vi "Begin.vi"(8 "error in":errorcluster) -> (0 "error out":errorcluster)   [LabVIEW 2019]
doc: "Called before other user functions, this VI is expected to open initial I/O refnums, load in file data, and do all program initialization. Notice that the <B>error out</B> terminal is simply used for data flow. Wiring it to other structures or subVIs ensures that this VI runs first."
uses:
  <vilib>/Rock Robotics/WPI/DriverStation/WPI_DriverStationRobotMode2.ctl
  Subsystems/Drive/Drive_Cluster.ctl
  Subsystems/Drive/Drive_States.ctl
  Subsystems/Intake/Intake_Cluster.ctl
  Subsystems/Intake/Intake_States.ctl
  Subsystems/Turret/Turret_Cluster.ctl
  Subsystems/Turret/Turret_States.ctl
  Subsystems/Magazine/Magazine_Cluster.ctl
  Subsystems/Magazine/Magazine_States.ctl
  Subsystems/Climb/Climb_Cluster.ctl
  Subsystems/Climb/Climb_States.ctl
  Subsystems/Control_Panel/Control_Panel_Cluster.ctl
  Subsystems/Control_Panel/Control_Panel_States.ctl
  <vilib>/Rock Robotics/WPI/Joystick/WPI_JoystickDeviceEnum.ctl
  Subsystems/Flywheel/Flywheel_Cluster.ctl
  Subsystems/Flywheel/Flywheel_States.ctl
  <vilib>/Rock Robotics/WPI/ThirdParty/REV Robotics/SPARK MAX/Typedef/Spark MAX Control Type.ctl
  <vilib>/Rock Robotics/WPI/ThirdParty/Phoenix-LabVIEW/Motor Controller/Controls/CTRE_Phoenix_MotorControl_ControlMode.ctl
  <vilib>/Rock Robotics/WPI/ThirdParty/REV Robotics/SPARK MAX/Typedef/Spark MAX Motor Type.ctl
  <vilib>/Rock Robotics/WPI/ThirdParty/REV Robotics/SPARK MAX/Typedef/Spark MAX Idle Mode.ctl
  <vilib>/Rock Robotics/WPI/ThirdParty/Phoenix-LabVIEW/Motor Controller/Controls/CTRE_Phoenix_MotorControl_SupplyCurrentLimitConfiguration.ctl
  <vilib>/Rock Robotics/WPI/ThirdParty/Phoenix-LabVIEW/Motor Controller/Controls/CTRE_Phoenix_MotorControl_TalonFXInvertType.ctl
  <vilib>/Rock Robotics/WPI/ThirdParty/Phoenix-LabVIEW/Motor Controller/Controls/CTRE_Phoenix_MotorControl_NeutralMode.ctl
  <vilib>/Rock Robotics/WPI/Solenoid/WPI_SolenoidChannel.ctl
  <vilib>/Rock Robotics/SystemInterfaces/AI/FPGA_AIChannel.ctl
  Robot Global Data.vi
  <vilib>/Rock Robotics/WPI/Solenoid/WPI_SolenoidOpenDouble.vi
  Globals/Drive_Globals.vi
  Globals/Intake_Globals.vi
  Globals/Turret_Globals.vi
  Globals/Magazine_Globals.vi
  Globals/Climb_Globals.vi
  Globals/Control_Panel_Globals.vi
  Globals/Joystick_Globals.vi
  Globals/Flywheel_Globals.vi
  Globals/Solenoid Globals.vi
  <vilib>/Rock Robotics/WPI/Utilities/WPI_GetSetVariantRefNum.vi
  <vilib>/Rock Robotics/WPI/ThirdParty/REV Robotics/SPARK MAX/Typedef/Spark MAX Sensor Type.ctl
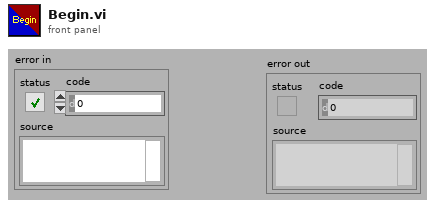
[diagram p1: front panel]
types:
  T1 = typedef "CTRE_Phoenix_MotorControl_NeutralMode.ctl" = enum8{"EEPROMSetting", "Override to Coast", "Override to Brake"}
  T2 = typedef "FPGA_AIChannel.ctl" = enum8{"AI 0", "AI 1", "AI 2", "AI 3", "AI MXP 0", "AI MXP 1", "AI MXP 2", "AI MXP 3", "Invalid"}
  T3 = typedef "WPI_SolenoidChannel.ctl" = enum8{"Solenoid 0", "Solenoid 1", "Solenoid 2", "Solenoid 3", "Solenoid 4", "Solenoid 5", "Solenoid 6", "Solenoid 7", "Invalid"}
  T4 = cluster{"P Gain":dbl, "I Gain":dbl, "D Gain":dbl, "F Gain":dbl, "I Zone":dbl, "Min Output":dbl, "Max Output":dbl}
  T5 = typedef "CTRE_Phoenix_MotorControl_TalonFXInvertType.ctl" = enum16{"Counter-Clockwise", "Clockwise"}
  T6 = typedef "CTRE_Phoenix_MotorControl_ControlMode.ctl" = u16
  T7 = typedef "CTRE_Phoenix_MotorControl_SupplyCurrentLimitConfiguration.ctl" = cluster{"Enable?":bool, "Current Limit":dbl, "Threshold Current":dbl, "Threshold Time":dbl}
  T8 = typedef "Spark MAX Idle Mode.ctl" = enum16{"Coast", "Brake"}
  T9 = typedef "Spark MAX Motor Type.ctl" = enum16{"Brushed", "Brushless"}
  T10 = typedef "Spark MAX Control Type.ctl" = enum16{"Percent VBus", "Voltage", "Velocity", "Position", "Smart Motion", "Current", "Smart Velocity"}
  T11 = typedef "Flywheel_Cluster.ctl" = cluster{"Flywheel_Throttle":dbl, "Control_States":T12, "Auto_Speed":bool, "Flywheel_On":bool, "Parameter_1":dbl, "Parameter_2":dbl, "Auto_Notifier":refnum<notifier>, "Step":dbl}
  T12 = typedef "Flywheel_States.ctl" = enum16{"No-Op", "Percent_Voltage", "Speed_Control_Manual", "Speed_Control_Auto"}
  T13 = typedef "WPI_JoystickDeviceEnum.ctl" = enum16{"USB 0", "USB 1", "USB 2", "USB 3", "USB 4", "USB 5"}
  T14 = typedef "Control_Panel_Cluster.ctl" = cluster{"Control_State":T15, "Start_Movement":bool, "Abort":bool, "Rotation_Control?":bool, "Positional_Control? ":bool, "Throttle":dbl}
  T15 = typedef "Control_Panel_States.ctl" = enum16{"No-Op", "Rotational_Control", "Positional_Control", "Manual_Control"}
  T16 = typedef "Climb_Cluster.ctl" = cluster{"Control_State":T17, "Extend_Climber?":bool, "Clamp?":bool, "Balance?":bool, "Transverse_Throttle":dbl, "Elevator_Throttle":dbl, "Control_Panel_Setpoint?":bool, "Auto-Balance":bool, "Pivot_Throttle":dbl}
  T17 = typedef "Climb_States.ctl" = enum16{"No-Op", "Extending", "Clamping", "Balancing", "Manual_Control"}
  T18 = typedef "Magazine_Cluster.ctl" = cluster{"Fire":bool, "Magazine_Throttle":dbl, "Control_States":T19, "Intake_Throttle":dbl, "Auto_Notifier":refnum<notifier>, "Parameter_1":dbl, "Parameter_2":dbl, "Step":dbl}
  T19 = typedef "Magazine_States.ctl" = enum16{"No-Op", "Loading", "Fire", "Unjam", "Manual_Percent_Voltage", "Manual_Speed_Control"}
  T20 = typedef "Turret_Cluster.ctl" = cluster{"Auto-Target?":bool, "Control_State":T21, "Turret_Spin_Speed":dbl, "Turret_Spin_Speed_Control?":bool}
  T21 = typedef "Turret_States.ctl" = enum16{"Manual_Percent_Voltage", "Manual_Speed_Control", "Auto-Target"}
  T22 = typedef "Intake_Cluster.ctl" = cluster{"Control_State":T23, "Intake_On":bool, "Intake_Extended":bool, "Intake_Throttle":dbl, "Auto_Notifier":refnum<notifier>, "Parameter_1":dbl, "Parameter_2":dbl, "Step":dbl}
  T23 = typedef "Intake_States.ctl" = enum16{"Manual_Control", "Compliant_Intake"}
  T24 = typedef "Drive_Cluster.ctl" = cluster{"Control_State":T25, "Angular_Throttle":dbl, "Linear_Throttle":dbl, "Torque_Changing":bool, "Step":dbl, "Parameter_1":dbl, "Parameter_2":dbl, "Parameter_3":dbl, "Parameter_4":dbl, "Auto_Notifier":refnum<notifier>}
  T25 = typedef "Drive_States.ctl" = enum16{"Percent_Voltage_Control", "Speed_Control"}
  T26 = typedef "WPI_DriverStationRobotMode2.ctl" = enum16{"Autonomous Disabled", "Autonomous Enabled", "Teleop Disabled", "Teleop Enabled", "Disconnected", "Finish", "Test Disabled", "Test Enabled", "Emergency Stopped"}
  T27 = typedef "WPI_AnalogChannelDevRef.ctl" = cluster{"DevStatus":errorcluster, "Analog Channel":T2}
  T28 = typedef "WPI_JoystickDevRef.ctl" = cluster{"Device":T13}
  T29 = typedef "WPI_MotorControlDeviceRef.ctl" = cluster{"DeviceStatus":errorcluster, "Type":T30, "PWM":cluster{"PWM Channel":T31, "DeadBand":T32}, "CAN":cluster{"Device Number":u8, "SetOutput VI Ref":variant, "GetOutput VI Ref":variant, "Enable VI Ref":variant, "Disable VI Ref":variant, "Data":variant}, "Invert":bool, "DIO PWM":cluster{"PWM \"Enable\" Channel":T31, "DIOChannel":T33, "PWM Rate":dbl}}
  T30 = typedef "WPI_MotorControlType.ctl" = enum16{"PWM", "CAN", "DIO PWM"}
  T31 = typedef "FPGA_DIOPWMChannel.ctl" = enum8{"PWM 0", "PWM 1", "PWM 2", "PWM 3", "PWM 4", "PWM 5", "PWM 6", "PWM 7", "PWM 8", "PWM 9", "PWM MXP 0", "PWM MXP 1", "PWM MXP 2", "PWM MXP 3", "PWM MXP 4", "PWM MXP 5", "PWM MXP 6", "PWM MXP 7", "PWM MXP 8", "PWM MXP 9", "Invalid"}
  T32 = typedef "WPI_PWMDeadband.ctl" = cluster{"Name":string, "maxPositivePwm":i32, "minPositivePwm":i32, "centerPwm":i32, "maxNegativePwm":i32, "minNegativePwm":i32, "angularRange":u16}
  T33 = typedef "FPGA_DIOChannel.ctl" = enum8{"DIO 0", "DIO 1", "DIO 2", "DIO 3", "DIO 4", "DIO 5", "DIO 6", "DIO 7", "DIO 8", "DIO 9", "DIO MXP 0", "DIO MXP 1", "DIO MXP 2", "DIO MXP 3", "DIO MXP 4", "DIO MXP 5", "DIO MXP 6", "DIO MXP 7", "DIO MXP 8", "DIO MXP 9", "DIO MXP 10", "DIO MXP 11", "DIO MXP 12", "DIO MXP 13", "DIO MXP 14", "DIO MXP 15", "SPI Port CS1", "SPI Port CS2", "SPI Port CS3", "SPI Port MISO", "SPI Port MOSI", "Invalid"}
  T34 = typedef "Spark MAX Sensor Type.ctl" = enum16{"No Sensor", "Hall Sensor", "Encoder", "-Not Available-", "Analog", "Alternate Encoder"}
  T35 = typedef "WPI_CompressorDevRef.ctl" = cluster{"DevStatus":errorcluster, "Pneumatics Control Module":u8}
  T36 = typedef "WPI_SolenoidDevRef.ctl" = cluster{"DevStatus":errorcluster, "Pneumatics Control Module":u8, "Forward Solenoid Channel":T3, "Reverse Solenoid Channel":T3}
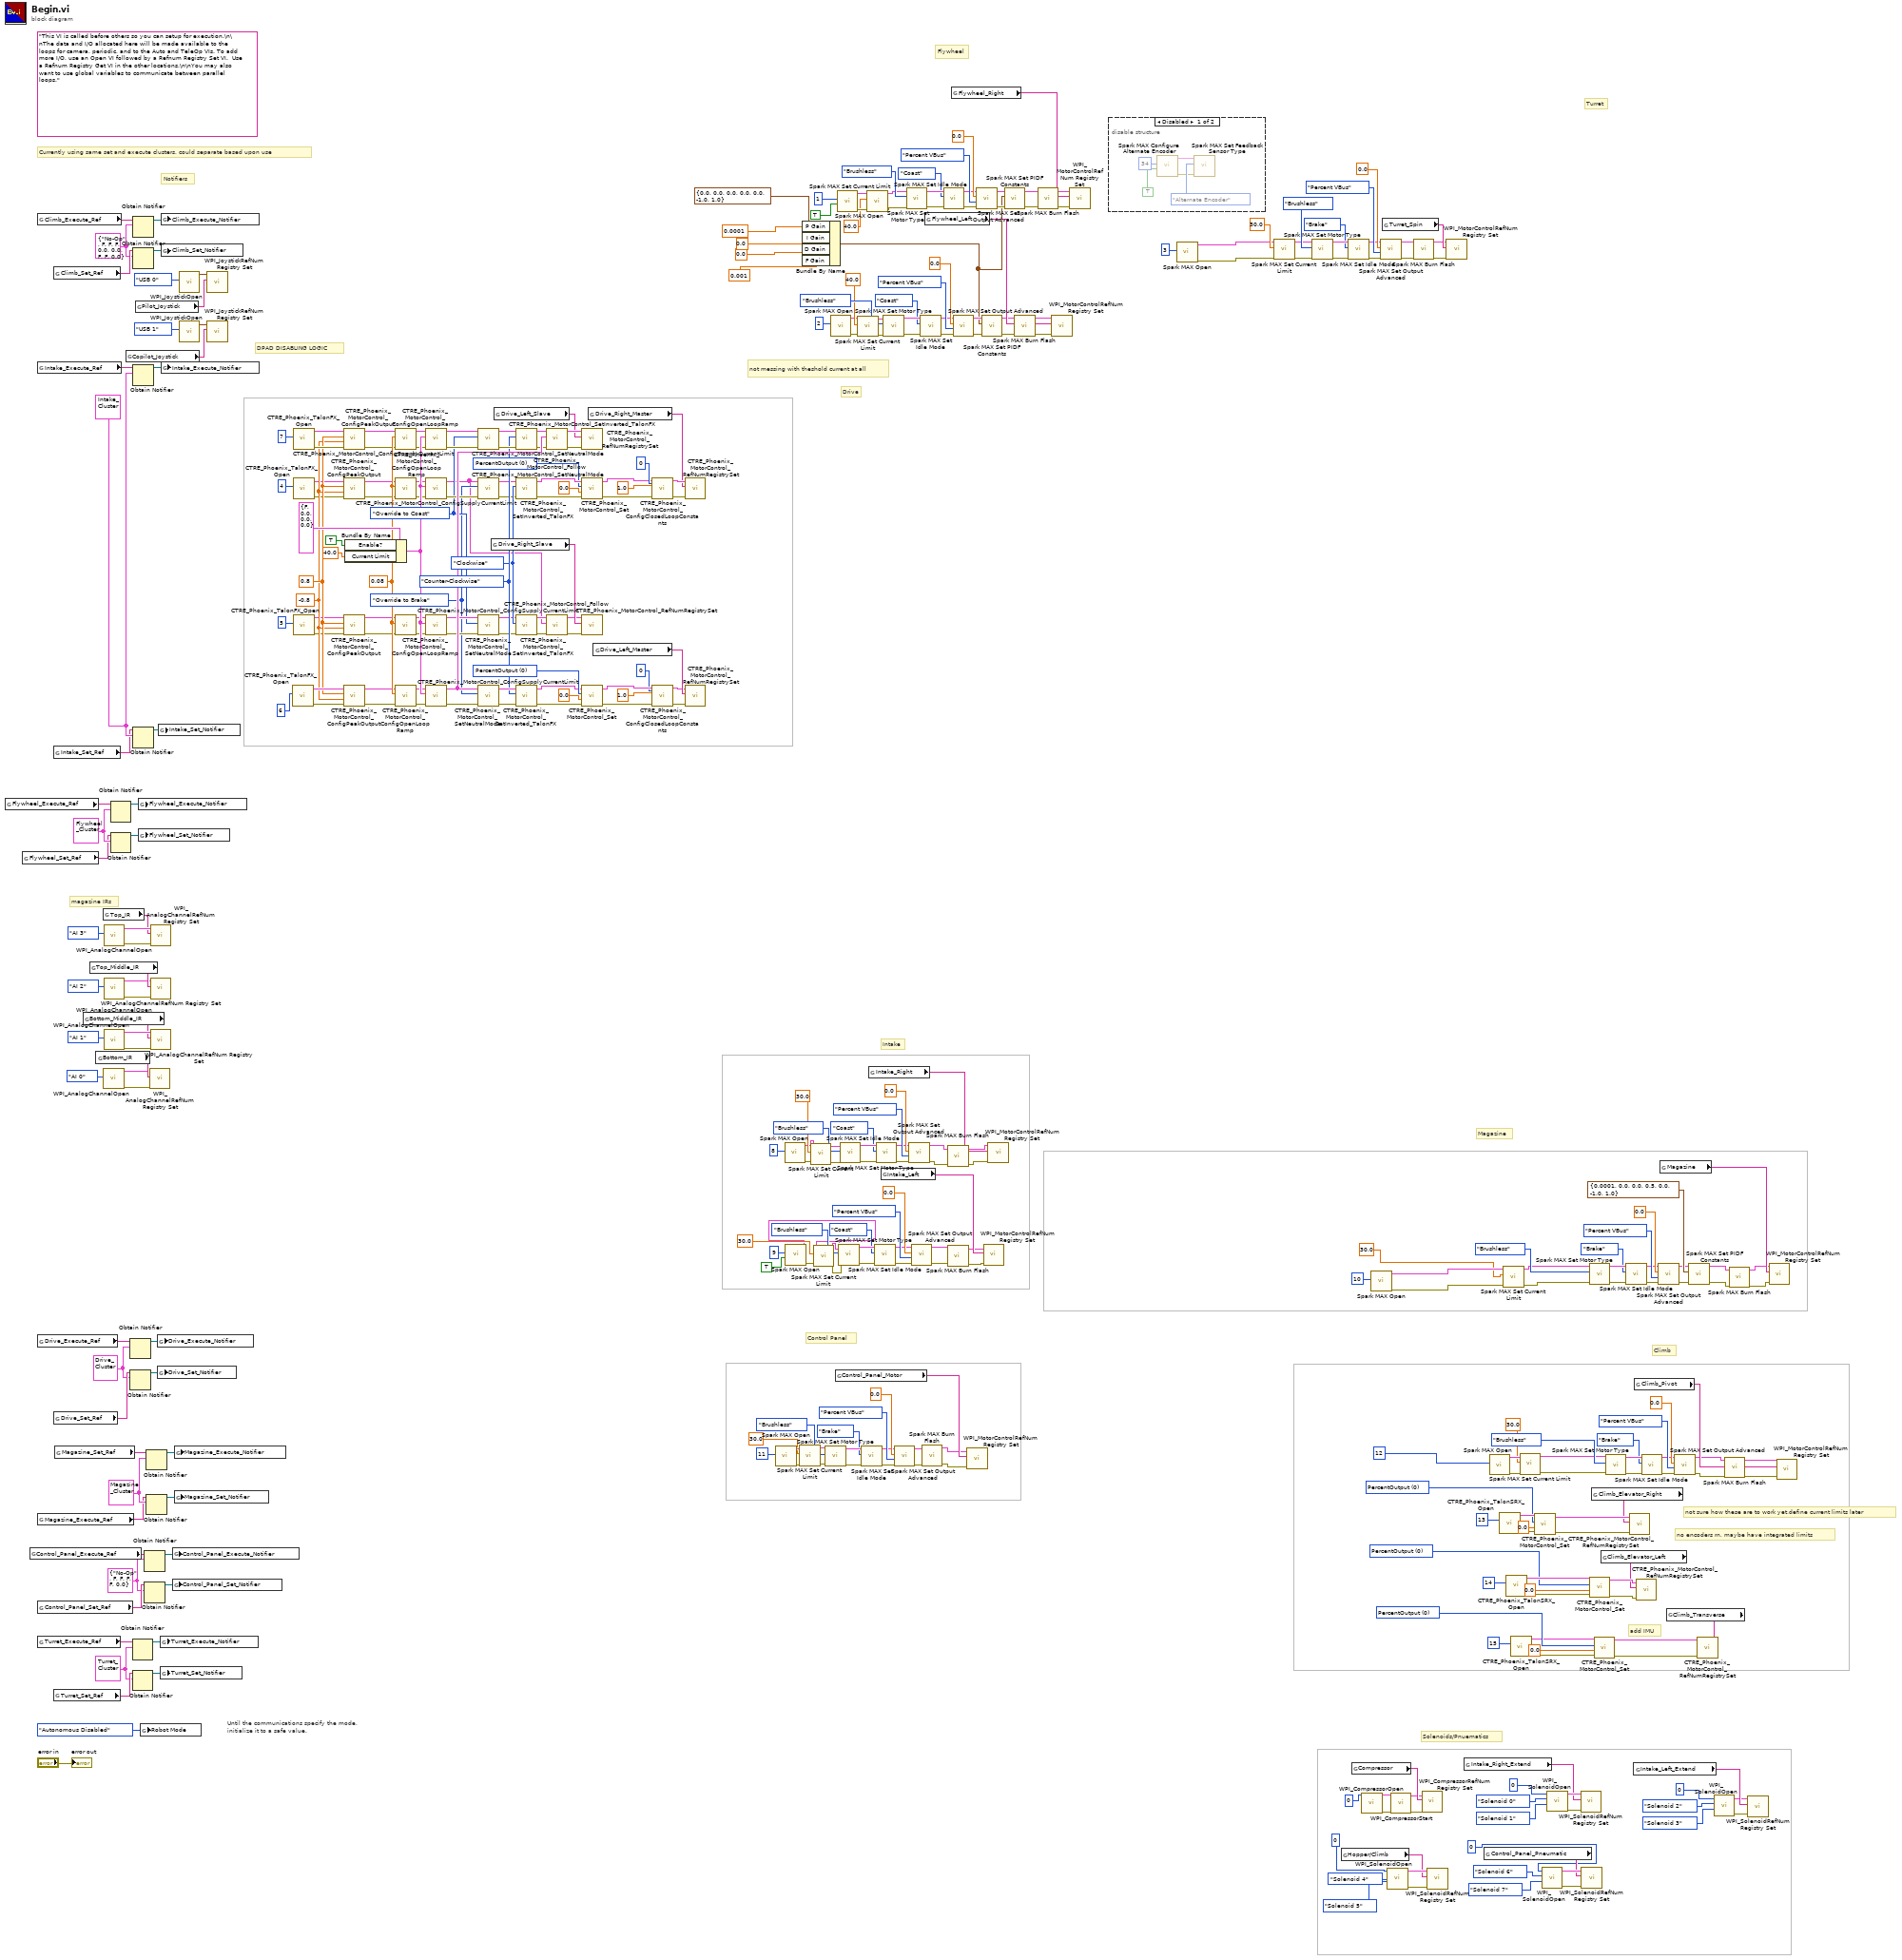
[diagram p0: block diagram]
diagram:
  w8 = CTRE_Phoenix_MotorControl_NeutralMode."Override to Brake" ("Motor Control Neutral Mode")
  w21 = -0.8 ("Forward Peak Percent Output")
  w22 = 0.8 ("Forward Peak Percent Output")
  w35 = 0.08 ("secondsFromNeutralToFull")
  w145 = CTRE_Phoenix_MotorControl_TalonFXInvertType."Clockwise" ("Invert Type")
  w120 = CTRE_Phoenix_MotorControl_NeutralMode."Override to Coast" ("Motor Control Neutral Mode")
  w126 = T6 0 items=["PercentOutput"=0, "Position"=1, "Velocity"=2, "Current"=3, "Follower"=5, "MotionProfile"=6, "MotionMagic"=7, "MotionProfileArc"=10, "Disabled"=15] ("Control Mode")
  w150 = CTRE_Phoenix_MotorControl_TalonFXInvertType."Counter-Clockwise" ("Invert Type")
  w254 = T6 0 items=["PercentOutput"=0, "Position"=1, "Velocity"=2, "Current"=3, "Follower"=5, "MotionProfile"=6, "MotionMagic"=7, "MotionProfileArc"=10, "Disabled"=15] ("Control Mode")
  w261 = T6 0 items=["PercentOutput"=0, "Position"=1, "Velocity"=2, "Current"=3, "Follower"=5, "MotionProfile"=6, "MotionMagic"=7, "MotionProfileArc"=10, "Disabled"=15] ("Control Mode")
  w270 = T6 0 items=["PercentOutput"=0, "Position"=1, "Velocity"=2, "Current"=3, "Follower"=5, "MotionProfile"=6, "MotionMagic"=7, "MotionProfileArc"=10, "Disabled"=15] ("Control Mode")
  w296 = T11 {"Flywheel_Throttle"=0.0, "Control_States"=enum."No-Op", "Auto_Speed"=FALSE, "Flywheel_On"=FALSE, "Parameter_1"=0.0, "Parameter_2"=0.0, "Auto_Notifier"=refnum, "Step"=0.0}
  w321 = T6 0 items=["PercentOutput"=0, "Position"=1, "Velocity"=2, "Current"=3, "Follower"=5, "MotionProfile"=6, "MotionMagic"=7, "MotionProfileArc"=10, "Disabled"=15] ("Control Mode")
  w348 = T14 {"Control_State"=enum."No-Op", "Start_Movement"=FALSE, "Abort"=FALSE, "Rotation_Control?"=FALSE, "Positional_Control? "=FALSE, "Throttle"=0.0}
  w352 = T16 {"Control_State"=enum."No-Op", "Extend_Climber?"=FALSE, "Clamp?"=FALSE, "Balance?"=FALSE, "Transverse_Throttle"=0.0, "Elevator_Throttle"=0.0, "Control_Panel_Setpoint?"=FALSE, "Auto-Balance"=FALSE, "Pivot_Throttle"=0.0}
  w356 = T18 {"Fire"=FALSE, "Magazine_Throttle"=0.0, "Control_States"=enum."No-Op", "Intake_Throttle"=0.0, "Auto_Notifier"=refnum, "Parameter_1"=0.0, "Parameter_2"=0.0, "Step"=0.0}
  w357 = T20 {"Auto-Target?"=FALSE, "Control_State"=enum."Manual_Percent_Voltage", "Turret_Spin_Speed"=0.0, "Turret_Spin_Speed_Control?"=FALSE}
  w362 = T22 {"Control_State"=enum."Manual_Control", "Intake_On"=FALSE, "Intake_Extended"=FALSE, "Intake_Throttle"=0.0, "Auto_Notifier"=refnum, "Parameter_1"=0.0, "Parameter_2"=0.0, "Step"=0.0}
  w363 = T24 {"Control_State"=enum."Percent_Voltage_Control", "Angular_Throttle"=0.0, "Linear_Throttle"=0.0, "Torque_Changing"=FALSE, "Step"=0.0, "Parameter_1"=0.0, "Parameter_2"=0.0, "Parameter_3"=0.0, "Parameter_4"=0.0, "Auto_Notifier"=refnum}
  (unwired) "This VI is called before others so you can setup for execution.\n\nThe data and I/O allocated here will be made available to the loops for camera, periodic, and to the Auto and TeleOp VIs. To add more I/O, use an Open VI followed by a Refnum Registry Set VI.  Use a Refnum Registry Get VI in the other locations.\n\nYou may also want to use global variables to communicate between parallel loops."
  # "magazine IRs"
  # "Solenoids/Pnuematics"
  # "not sure how these are to work yet,define current limits later"
  # "not messing with theshold current at all"
  # "add IMU"
  # "no encoders rn, maybe have integrated limits"
  # "Climb"
  # "Control Panel"
  # "Magazine"
  # "Intake"
  # "Drive"
  # "Turret"
  # "Flywheel"
  # "DPAD DISABLING LOGIC"
  # "Notifiers"
  # "Currently using same set and execute clusters, could separate based upon use"
  # "Until the communications specify the mode,\ninitialize it to a safe value."
  n1 = global read "Flywheel_Globals.vi" "Flywheel_Execute_Ref"() -> (w295:string)
  n2 = global read "Flywheel_Globals.vi" "Flywheel_Set_Ref"() -> (w294:string)
  n3 = global read "Control_Panel_Globals.vi" "Control_Panel_Execute_Ref"() -> (w350:string)
  n4 = global read "Climb_Globals.vi" "Climb_Execute_Ref"() -> (w351:string)
  n5 = global read "Intake_Globals.vi" "Intake_Execute_Ref"() -> (w361:string)
  n6 = global read "Drive_Globals.vi" "Drive_Execute_Ref"() -> (w364:string)
  n7 = global read "Magazine_Globals.vi" "Magazine_Execute_Ref"() -> (w355:string)
  n8 = global read "Control_Panel_Globals.vi" "Control_Panel_Set_Ref"() -> (w349:string)
  n9 = global read "Turret_Globals.vi" "Turret_Execute_Ref"() -> (w359:string)
  n10 = global read "Climb_Globals.vi" "Climb_Set_Ref"() -> (w353:string)
  n11 = global read "Intake_Globals.vi" "Intake_Set_Ref"() -> (w360:string)
  n12 = global read "Drive_Globals.vi" "Drive_Set_Ref"() -> (w365:string)
  n13 = global read "Turret_Globals.vi" "Turret_Set_Ref"() -> (w358:string)
  n14 = global read "Magazine_Globals.vi" "Magazine_Set_Ref"() -> (w354:string)
  n15 = global read "Magazine_Globals.vi" "Bottom_Middle_IR"() -> (w40:string)
  n16 = global read "Magazine_Globals.vi" "Top_Middle_IR"() -> (w47:string)
  n17 = global read "Magazine_Globals.vi" "Bottom_IR"() -> (w39:string)
  n18 = global read "Magazine_Globals.vi" "Top_IR"() -> (w48:string)
  n19 = call <vilib>:"WPI_AnalogChannelOpen.vi"("Analog Channel"=FPGA_AIChannel."AI 0") -> ("error out"=w38:errorcluster, "AIDeviceRef"=w37:T27)  [unwired: 9 in]
  n20 = call <vilib>:"WPI_AnalogChannelOpen.vi"("Analog Channel"=FPGA_AIChannel."AI 3") -> ("error out"=w49:errorcluster, "AIDeviceRef"=w50:T27)  [unwired: 9 in]
  n21 = call <vilib>:"WPI_AnalogChannelOpen.vi"("Analog Channel"=FPGA_AIChannel."AI 2") -> ("error out"=w46:errorcluster, "AIDeviceRef"=w45:T27)  [unwired: 9 in]
  n22 = call <vilib>:"WPI_AnalogChannelOpen.vi"("Analog Channel"=FPGA_AIChannel."AI 1") -> ("error out"=w41:errorcluster, "AIDeviceRef"=w42:T27)  [unwired: 9 in]
  n23 = Obtain Notifier(name (unnamed)=w295, notification data type=w296) -> (notifier out=w292:refnum<notifier>)  [unwired: 2 in, 2 out]
  n24 = Obtain Notifier(name (unnamed)=w294, notification data type=w296) -> (notifier out=w293:refnum<notifier>)  [unwired: 2 in, 2 out]
  n25 = global read "Joystick_Globals.vi" "Copilot_Joystick"() -> (w330:string)
  n26 = Obtain Notifier(name (unnamed)=w364, notification data type=w363) -> (notifier out=w342:refnum<notifier>)  [unwired: 2 in, 2 out]
  n27 = Obtain Notifier(name (unnamed)=w365, notification data type=w363) -> (notifier out=w343:refnum<notifier>)  [unwired: 2 in, 2 out]
  n28 = Obtain Notifier(name (unnamed)=w359, notification data type=w357) -> (notifier out=w336:refnum<notifier>)  [unwired: 2 in, 2 out]
  n29 = Obtain Notifier(name (unnamed)=w358, notification data type=w357) -> (notifier out=w337:refnum<notifier>)  [unwired: 2 in, 2 out]
  n30 = Obtain Notifier(name (unnamed)=w351, notification data type=w352) -> (notifier out=w346:refnum<notifier>)  [unwired: 2 in, 2 out]
  n31 = Obtain Notifier(name (unnamed)=w353, notification data type=w352) -> (notifier out=w347:refnum<notifier>)  [unwired: 2 in, 2 out]
  n32 = Obtain Notifier(name (unnamed)=w361, notification data type=w362) -> (notifier out=w344:refnum<notifier>)  [unwired: 2 in, 2 out]
  n33 = Obtain Notifier(name (unnamed)=w360, notification data type=w362) -> (notifier out=w345:refnum<notifier>)  [unwired: 2 in, 2 out]
  n34 = global read "Joystick_Globals.vi" "Pilot_Joystick"() -> (w331:string)
  n35 = global write "Flywheel_Globals.vi" "Flywheel_Execute_Notifier"(w292) -> ()
  n36 = global write "Flywheel_Globals.vi" "Flywheel_Set_Notifier"(w293) -> ()
  n37 = global write "Robot Global Data.vi" "Robot Mode"(WPI_DriverStationRobotMode2."Autonomous Disabled" ("Robot Mode")) -> ()
  n38 = Obtain Notifier(name (unnamed)=w350, notification data type=w348) -> (notifier out=w338:refnum<notifier>)  [unwired: 2 in, 2 out]
  n39 = Obtain Notifier(name (unnamed)=w349, notification data type=w348) -> (notifier out=w339:refnum<notifier>)  [unwired: 2 in, 2 out]
  n40 = Obtain Notifier(name (unnamed)=w354, notification data type=w356) -> (notifier out=w340:refnum<notifier>)  [unwired: 2 in, 2 out]
  n41 = Obtain Notifier(name (unnamed)=w355, notification data type=w356) -> (notifier out=w341:refnum<notifier>)  [unwired: 2 in, 2 out]
  n42 = call <vilib>:"WPI_AnalogChannelRefNum Registry Set.vi"("error in (no error)"=w38, "refnum name"=w39, "AIDeviceRef"=w37) -> ()  [unwired: 7 in, 2 out]
  n43 = call <vilib>:"WPI_AnalogChannelRefNum Registry Set.vi"("error in (no error)"=w49, "refnum name"=w48, "AIDeviceRef"=w50) -> ()  [unwired: 7 in, 2 out]
  n44 = call <vilib>:"WPI_AnalogChannelRefNum Registry Set.vi"("error in (no error)"=w46, "refnum name"=w47, "AIDeviceRef"=w45) -> ()  [unwired: 7 in, 2 out]
  n45 = call <vilib>:"WPI_AnalogChannelRefNum Registry Set.vi"("error in (no error)"=w41, "refnum name"=w40, "AIDeviceRef"=w42) -> ()  [unwired: 7 in, 2 out]
  n46 = global write "Drive_Globals.vi" "Drive_Execute_Notifier"(w342) -> ()
  n47 = global write "Drive_Globals.vi" "Drive_Set_Notifier"(w343) -> ()
  n48 = global write "Intake_Globals.vi" "Intake_Set_Notifier"(w345) -> ()
  n49 = global write "Turret_Globals.vi" "Turret_Execute_Notifier"(w336) -> ()
  n50 = global write "Turret_Globals.vi" "Turret_Set_Notifier"(w337) -> ()
  n51 = global write "Climb_Globals.vi" "Climb_Execute_Notifier"(w346) -> ()
  n52 = global write "Climb_Globals.vi" "Climb_Set_Notifier"(w347) -> ()
  n53 = global write "Intake_Globals.vi" "Intake_Execute_Notifier"(w344) -> ()
  n54 = global write "Control_Panel_Globals.vi" "Control_Panel_Execute_Notifier"(w338) -> ()
  n55 = global write "Control_Panel_Globals.vi" "Control_Panel_Set_Notifier"(w339) -> ()
  n56 = global write "Magazine_Globals.vi" "Magazine_Execute_Notifier"(w340) -> ()
  n57 = global write "Magazine_Globals.vi" "Magazine_Set_Notifier"(w341) -> ()
  n58 = call <vilib>:"WPI_JoystickOpen.vi"("JoystickDevice"=WPI_JoystickDeviceEnum."USB 0") -> ("JoystickDevRef"=w335:T28)  [unwired: 10 in]
  n59 = call <vilib>:"WPI_JoystickOpen.vi"("JoystickDevice"=WPI_JoystickDeviceEnum."USB 1") -> ("JoystickDevRef"=w334:T28)  [unwired: 10 in]
  n60 = call <vilib>:"WPI_JoystickRefNum Registry Set.vi"("refnum name"=w331, "JoystickDevRef"=w335) -> ()  [unwired: 8 in, 2 out]
  n61 = call <vilib>:"WPI_JoystickRefNum Registry Set.vi"("refnum name"=w330, "JoystickDevRef"=w334) -> ()  [unwired: 8 in, 2 out]
  n62 = call <vilib>:"CTRE_Phoenix_TalonFX_Open.vi"("Device Number"=u8 6) -> ("error out"=w23:errorcluster, "CAN Talon SRX Ref"=w24:T29)  [unwired: 9 in]
  n63 = call <vilib>:"CTRE_Phoenix_TalonFX_Open.vi"("Device Number"=u8 7) -> ("error out"=w34:errorcluster, "CAN Talon SRX Ref"=w33:T29)  [unwired: 9 in]
  n64 = call <vilib>:"CTRE_Phoenix_TalonFX_Open.vi"("Device Number"=u8 4) -> ("error out"=w19:errorcluster, "CAN Talon SRX Ref"=w20:T29)  [unwired: 9 in]
  n65 = call <vilib>:"CTRE_Phoenix_TalonFX_Open.vi"("Device Number"=u8 5) -> ("error out"=w17:errorcluster, "CAN Talon SRX Ref"=w18:T29)  [unwired: 9 in]
  n66 = call <vilib>:"CTRE_Phoenix_MotorControl_ConfigPeakOutput.vi"("error in (no error)"=w34, "Reverse Peak Percent Output"=w21, "Forward Peak Percent Output"=w22, "PhoenixMotorControlDevRef"=w33) -> ("error out"=w31:errorcluster, "PhoenixMotorControlDevRef"=w32:T29)  [unwired: 6 in]
  n67 = call <vilib>:"CTRE_Phoenix_MotorControl_ConfigPeakOutput.vi"("error in (no error)"=w19, "Reverse Peak Percent Output"=w21, "Forward Peak Percent Output"=w22, "PhoenixMotorControlDevRef"=w20) -> ("error out"=w30:errorcluster, "PhoenixMotorControlDevRef"=w29:T29)  [unwired: 6 in]
  n68 = call <vilib>:"CTRE_Phoenix_MotorControl_ConfigPeakOutput.vi"("error in (no error)"=w17, "Reverse Peak Percent Output"=w21, "Forward Peak Percent Output"=w22, "PhoenixMotorControlDevRef"=w18) -> ("error out"=w28:errorcluster, "PhoenixMotorControlDevRef"=w27:T29)  [unwired: 6 in]
  n69 = call <vilib>:"CTRE_Phoenix_MotorControl_ConfigPeakOutput.vi"("error in (no error)"=w23, "Reverse Peak Percent Output"=w21, "Forward Peak Percent Output"=w22, "PhoenixMotorControlDevRef"=w24) -> ("error out"=w26:errorcluster, "PhoenixMotorControlDevRef"=w25:T29)  [unwired: 6 in]
  n70 = Bundle By Name(cluster=T7 {"Enable?"=FALSE, "Current Limit"=0.0, "Threshold Current"=0.0, "Threshold Time"=0.0} ("Supply Current Limit Configuration"), "Enable?"=TRUE, "Current Limit"=40.0) -> (w121:T7)
  n71 = call <vilib>:"CTRE_Phoenix_MotorControl_ConfigOpenLoopRamp.vi"("error in (no error)"=w31, "secondsFromNeutralToFull"=w35, "PhoenixMotorControlDevRef"=w32) -> ("error out"=w9:errorcluster, "PhoenixMotorControlDevRef"=w10:T29)  [unwired: 7 in]
  n72 = call <vilib>:"CTRE_Phoenix_MotorControl_ConfigOpenLoopRamp.vi"("error in (no error)"=w30, "secondsFromNeutralToFull"=w35, "PhoenixMotorControlDevRef"=w29) -> ("error out"=w11:errorcluster, "PhoenixMotorControlDevRef"=w12:T29)  [unwired: 7 in]
  n73 = call <vilib>:"CTRE_Phoenix_MotorControl_ConfigOpenLoopRamp.vi"("error in (no error)"=w28, "secondsFromNeutralToFull"=w35, "PhoenixMotorControlDevRef"=w27) -> ("error out"=w15:errorcluster, "PhoenixMotorControlDevRef"=w16:T29)  [unwired: 7 in]
  n74 = call <vilib>:"CTRE_Phoenix_MotorControl_ConfigOpenLoopRamp.vi"("error in (no error)"=w26, "secondsFromNeutralToFull"=w35, "PhoenixMotorControlDevRef"=w25) -> ("error out"=w13:errorcluster, "PhoenixMotorControlDevRef"=w14:T29)  [unwired: 7 in]
  n75 = call <vilib>:"CTRE_Phoenix_MotorControl_ConfigSupplyCurrentLimit.vi"("error in (no error)"=w9, "Supply Current Limit Configuration"=w121, "PhoenixMotorControlDevRef"=w10) -> ("error out"=w158:errorcluster, "PhoenixMotorControlDevRef"=w159:T29)  [unwired: 7 in]
  n76 = call <vilib>:"CTRE_Phoenix_MotorControl_ConfigSupplyCurrentLimit.vi"("error in (no error)"=w11, "Supply Current Limit Configuration"=w121, "PhoenixMotorControlDevRef"=w12) -> ("error out"=w136:errorcluster, "PhoenixMotorControlDevRef"=w7:T29)  [unwired: 7 in]
  n77 = call <vilib>:"CTRE_Phoenix_MotorControl_ConfigSupplyCurrentLimit.vi"("error in (no error)"=w15, "Supply Current Limit Configuration"=w121, "PhoenixMotorControlDevRef"=w16) -> ("error out"=w138:errorcluster, "PhoenixMotorControlDevRef"=w137:T29)  [unwired: 7 in]
  n78 = call <vilib>:"CTRE_Phoenix_MotorControl_ConfigSupplyCurrentLimit.vi"("error in (no error)"=w13, "Supply Current Limit Configuration"=w121, "PhoenixMotorControlDevRef"=w14) -> ("error out"=w160:errorcluster, "PhoenixMotorControlDevRef"=w155:T29)  [unwired: 7 in]
  n79 = call <vilib>:"CTRE_Phoenix_MotorControl_SetNeutralMode.vi"("error in (no error)"=w158, "Motor Control Neutral Mode"=w120, "PhoenixMotorControlDevRef"=w159) -> ("error out"=w153:errorcluster, "PhoenixMotorControlDevRef"=w154:T29)  [unwired: 7 in]
  n80 = call <vilib>:"CTRE_Phoenix_MotorControl_SetNeutralMode.vi"("error in (no error)"=w136, "Motor Control Neutral Mode"=w8, "PhoenixMotorControlDevRef"=w7) -> ("error out"=w139:errorcluster, "PhoenixMotorControlDevRef"=w140:T29)  [unwired: 7 in]
  n81 = call <vilib>:"CTRE_Phoenix_MotorControl_SetNeutralMode.vi"("error in (no error)"=w138, "Motor Control Neutral Mode"=w120, "PhoenixMotorControlDevRef"=w137) -> ("error out"=w142:errorcluster, "PhoenixMotorControlDevRef"=w141:T29)  [unwired: 7 in]
  n82 = call <vilib>:"CTRE_Phoenix_MotorControl_SetNeutralMode.vi"("error in (no error)"=w160, "Motor Control Neutral Mode"=w8, "PhoenixMotorControlDevRef"=w155) -> ("error out"=w157:errorcluster, "PhoenixMotorControlDevRef"=w156:T29)  [unwired: 7 in]
  n83 = global read "Drive_Globals.vi" "Drive_Right_Slave"() -> (w127:string)
  n84 = global read "Drive_Globals.vi" "Drive_Left_Slave"() -> (w320:string)
  n85 = call <vilib>:"CTRE_Phoenix_MotorControl_SetInverted_TalonFX.vi"("error in (no error)"=w153, "Invert Type"=w150, "PhoenixMotorControlDevRef"=w154) -> ("error out"=w152:errorcluster, "PhoenixMotorControlDevRef"=w151:T29)  [unwired: 7 in]
  n86 = call <vilib>:"CTRE_Phoenix_MotorControl_SetInverted_TalonFX.vi"("error in (no error)"=w139, "Invert Type"=w145, "PhoenixMotorControlDevRef"=w140) -> ("error out"=w146:errorcluster, "PhoenixMotorControlDevRef"=w147:T29)  [unwired: 7 in]
  n87 = call <vilib>:"CTRE_Phoenix_MotorControl_SetInverted_TalonFX.vi"("error in (no error)"=w142, "Invert Type"=w145, "PhoenixMotorControlDevRef"=w141) -> ("error out"=w143:errorcluster, "PhoenixMotorControlDevRef"=w144:T29)  [unwired: 7 in]
  n88 = call <vilib>:"CTRE_Phoenix_MotorControl_SetInverted_TalonFX.vi"("error in (no error)"=w157, "Invert Type"=w150, "PhoenixMotorControlDevRef"=w156) -> ("error out"=w149:errorcluster, "PhoenixMotorControlDevRef"=w148:T29)  [unwired: 7 in]
  n89 = call <vilib>:"CTRE_Phoenix_MotorControl_Follow.vi"("error in (no error)"=w152, "Master Controller to Follow"=w155, "PhoenixMotorControlDevRef"=w151) -> ("error out"=w325:errorcluster, "PhoenixMotorControlDevRef"=w324:T29)  [unwired: 7 in]
  n90 = call <vilib>:"CTRE_Phoenix_MotorControl_Follow.vi"("error in (no error)"=w143, "Master Controller to Follow"=w7, "PhoenixMotorControlDevRef"=w144) -> ("error out"=w122:errorcluster, "PhoenixMotorControlDevRef"=w123:T29)  [unwired: 7 in]
  n91 = call <vilib>:"CTRE_Phoenix_MotorControl_RefNumRegistrySet.vi"("error in (no error)"=w325, "refnum name"=w320, "PhoenixMotorControlDevRef"=w324) -> ()  [unwired: 7 in, 2 out]
  n92 = call <vilib>:"CTRE_Phoenix_MotorControl_Set.vi"("error in (no error)"=w146, "Output"=0.0, "Control Mode"=w126, "PhoenixMotorControlDevRef"=w147) -> ("error out"=w131:errorcluster, "PhoenixMotorControlDevRef"=w130:T29)  [unwired: 6 in]
  n93 = call <vilib>:"CTRE_Phoenix_MotorControl_RefNumRegistrySet.vi"("error in (no error)"=w122, "refnum name"=w127, "PhoenixMotorControlDevRef"=w123) -> ()  [unwired: 7 in, 2 out]
  n94 = call <vilib>:"CTRE_Phoenix_MotorControl_Set.vi"("error in (no error)"=w149, "Output"=0.0, "Control Mode"=w321, "PhoenixMotorControlDevRef"=w148) -> ("error out"=w316:errorcluster, "PhoenixMotorControlDevRef"=w317:T29)  [unwired: 6 in]
  n95 = global read "Drive_Globals.vi" "Drive_Right_Master"() -> (w124:string)
  n96 = global read "Drive_Globals.vi" "Drive_Left_Master"() -> (w323:string)
  n97 = call <vilib>:"CTRE_Phoenix_MotorControl_ConfigClosedLoopConstants.vi"("PhoenixMotorControlDevRef"=w130, "slotIdx"=0, "P"=1.0, "error in (no error)"=w131) -> ("PhoenixMotorControlDevRef"=w134:T29, "error out"=w135:errorcluster)  [unwired: 10 in]
  n98 = call <vilib>:"CTRE_Phoenix_MotorControl_ConfigClosedLoopConstants.vi"("PhoenixMotorControlDevRef"=w317, "slotIdx"=0, "P"=1.0, "error in (no error)"=w316) -> ("PhoenixMotorControlDevRef"=w249:T29, "error out"=w248:errorcluster)  [unwired: 10 in]
  n99 = call <vilib>:"CTRE_Phoenix_MotorControl_RefNumRegistrySet.vi"("error in (no error)"=w135, "refnum name"=w124, "PhoenixMotorControlDevRef"=w134) -> ()  [unwired: 7 in, 2 out]
  n100 = call <vilib>:"CTRE_Phoenix_MotorControl_RefNumRegistrySet.vi"("error in (no error)"=w248, "refnum name"=w323, "PhoenixMotorControlDevRef"=w249) -> ()  [unwired: 7 in, 2 out]
  n101 = call <vilib>:"Spark MAX Open.vi"("Device Number"=u8 11) -> ("error out"=w168:errorcluster, "MotorControlDeviceRef"=w167:T29)  [unwired: 9 in]
  n102 = call <vilib>:"Spark MAX Open.vi"("Device Number"=u8 8) -> ("error out"=w180:errorcluster, "MotorControlDeviceRef"=w117:T29)  [unwired: 9 in]
  n103 = call <vilib>:"Spark MAX Open.vi"("Invert"=TRUE, "Device Number"=u8 9) -> ("error out"=w174:errorcluster, "MotorControlDeviceRef"=w118:T29)  [unwired: 8 in]
  n104 = call <vilib>:"Spark MAX Set Current Limit.vi"("error in (no error)"=w168, "Current Limit A (100)"=sgl 30.0, "MotorControlDeviceRef in"=w167) -> ("error out"=w165:errorcluster, "MotorControlDeviceRef out"=w166:T29)  [unwired: 7 in]
  n105 = Bundle By Name(cluster=T4 {"P Gain"=0.0, "I Gain"=0.0, "D Gain"=0.0, "F Gain"=0.0, "I Zone"=0.0, "Min Output"=-1.0, "Max Output"=1.0} ("PID Constants"), "P Gain"=0.0001, "I Gain"=0.0, "D Gain"=0.0, "F Gain"=0.001) -> (w5:T4)
  n106 = call <vilib>:"Spark MAX Set Current Limit.vi"("error in (no error)"=w180, "Current Limit A (100)"=sgl 30.0, "MotorControlDeviceRef in"=w117) -> ("error out"=w178:errorcluster, "MotorControlDeviceRef out"=w179:T29)  [unwired: 7 in]
  n107 = call <vilib>:"Spark MAX Set Current Limit.vi"("error in (no error)"=w174, "Current Limit A (100)"=sgl 30.0, "MotorControlDeviceRef in"=w118) -> ("error out"=w176:errorcluster, "MotorControlDeviceRef out"=w175:T29)  [unwired: 7 in]
  n108 = call <vilib>:"Spark MAX Set Motor Type.vi"("error in (no error)"=w165, "Motor Type"=Spark_MAX_Motor_Type."Brushless", "MotorControlDevRef"=w166) -> ("error out"=w205:errorcluster, "MotorControlDeviceRef"=w202:T29)  [unwired: 7 in]
  n109 = call <vilib>:"Spark MAX Open.vi"("Device Number"=u8 2) -> ("error out"=w187:errorcluster, "MotorControlDeviceRef"=w186:T29)  [unwired: 9 in]
  n110 = global read "Control_Panel_Globals.vi" "Control_Panel_Motor"() -> (w278:string)
  n111 = call <vilib>:"Spark MAX Open.vi"("Invert"=TRUE, "Device Number"=u8 1) -> ("error out"=w193:errorcluster, "MotorControlDeviceRef"=w192:T29)  [unwired: 8 in]
  n112 = call <vilib>:"Spark MAX Set Motor Type.vi"("error in (no error)"=w176, "Motor Type"=Spark_MAX_Motor_Type."Brushless", "MotorControlDevRef"=w175) -> ("error out"=w223:errorcluster, "MotorControlDeviceRef"=w220:T29)  [unwired: 7 in]
  n113 = call <vilib>:"Spark MAX Set Motor Type.vi"("error in (no error)"=w178, "Motor Type"=Spark_MAX_Motor_Type."Brushless", "MotorControlDevRef"=w179) -> ("error out"=w229:errorcluster, "MotorControlDeviceRef"=w228:T29)  [unwired: 7 in]
  n114 = call <vilib>:"Spark MAX Set Current Limit.vi"("error in (no error)"=w187, "Current Limit A (100)"=sgl 40.0, "MotorControlDeviceRef in"=w186) -> ("error out"=w184:errorcluster, "MotorControlDeviceRef out"=w185:T29)  [unwired: 7 in]
  n115 = call <vilib>:"Spark MAX Set Idle Mode.vi"("error in (no error)"=w205, "Idle Mode"=Spark_MAX_Idle_Mode."Brake", "MotorControlDeviceRef in"=w202) -> ("error out"=w204:errorcluster, "MotorControlDeviceRef out"=w203:T29)  [unwired: 7 in]
  n116 = call <vilib>:"Spark MAX Set Current Limit.vi"("error in (no error)"=w193, "Current Limit A (100)"=sgl 40.0, "MotorControlDeviceRef in"=w192) -> ("error out"=w191:errorcluster, "MotorControlDeviceRef out"=w190:T29)  [unwired: 7 in]
  n117 = global read "Intake_Globals.vi" "Intake_Right"() -> (w298:string)
  n118 = call <vilib>:"Spark MAX Set Idle Mode.vi"("error in (no error)"=w223, "Idle Mode"=Spark_MAX_Idle_Mode."Coast", "MotorControlDeviceRef in"=w220) -> ("error out"=w222:errorcluster, "MotorControlDeviceRef out"=w221:T29)  [unwired: 7 in]
  n119 = call <vilib>:"Spark MAX Set Idle Mode.vi"("error in (no error)"=w229, "Idle Mode"=Spark_MAX_Idle_Mode."Coast", "MotorControlDeviceRef in"=w228) -> ("error out"=w226:errorcluster, "MotorControlDeviceRef out"=w227:T29)  [unwired: 7 in]
  n120 = global read "Intake_Globals.vi" "Intake_Left"() -> (w297:string)
  n121 = call <vilib>:"Spark MAX Set Motor Type.vi"("error in (no error)"=w184, "Motor Type"=Spark_MAX_Motor_Type."Brushless", "MotorControlDevRef"=w185) -> ("error out"=w241:errorcluster, "MotorControlDeviceRef"=w240:T29)  [unwired: 7 in]
  n122 = call <vilib>:"Spark MAX Set Output Advanced.vi"("error in (no error)"=w204, "Control Mode"=Spark_MAX_Control_Type."Percent VBus", "Setpoint"=0.0, "MotorControlDevRef"=w203) -> ("error out"=w88:errorcluster, "MotorControlDevRef"=w89:T29)  [unwired: 6 in]
  n123 = call <vilib>:"Spark MAX Set Motor Type.vi"("error in (no error)"=w191, "Motor Type"=Spark_MAX_Motor_Type."Brushless", "MotorControlDevRef"=w190) -> ("error out"=w246:errorcluster, "MotorControlDeviceRef"=w247:T29)  [unwired: 7 in]
  n124 = call <vilib>:"Spark MAX Set Output Advanced.vi"("error in (no error)"=w226, "Control Mode"=Spark_MAX_Control_Type."Percent VBus", "Setpoint"=0.0, "MotorControlDevRef"=w227) -> ("error out"=w94:errorcluster, "MotorControlDevRef"=w95:T29)  [unwired: 6 in]
  n125 = call <vilib>:"Spark MAX Set Output Advanced.vi"("error in (no error)"=w222, "Control Mode"=Spark_MAX_Control_Type."Percent VBus", "Setpoint"=0.0, "MotorControlDevRef"=w221) -> ("error out"=w90:errorcluster, "MotorControlDevRef"=w91:T29)  [unwired: 6 in]
  n126 = call <vilib>:"Spark MAX Set Idle Mode.vi"("error in (no error)"=w241, "Idle Mode"=Spark_MAX_Idle_Mode."Coast", "MotorControlDeviceRef in"=w240) -> ("error out"=w239:errorcluster, "MotorControlDeviceRef out"=w238:T29)  [unwired: 7 in]
  n127 = call <vilib>:"Spark MAX Burn Flash.vi"("error in"=w88, "MotorControlDeviceRef"=w89) -> ("error out"=w86:errorcluster, "MotorControlDeviceRef"=w87:T29)  [unwired: 8 in]
  n128 = global read "Flywheel_Globals.vi" "Flywheel_Left"() -> (w328:string)
  n129 = call <vilib>:"Spark MAX Set Idle Mode.vi"("error in (no error)"=w246, "Idle Mode"=Spark_MAX_Idle_Mode."Coast", "MotorControlDeviceRef in"=w247) -> ("error out"=w242:errorcluster, "MotorControlDeviceRef out"=w243:T29)  [unwired: 7 in]
  n130 = call <vilib>:"Spark MAX Burn Flash.vi"("error in"=w94, "MotorControlDeviceRef"=w95) -> ("error out"=w97:errorcluster, "MotorControlDeviceRef"=w96:T29)  [unwired: 8 in]
  n131 = call <vilib>:"Spark MAX Burn Flash.vi"("error in"=w90, "MotorControlDeviceRef"=w91) -> ("error out"=w93:errorcluster, "MotorControlDeviceRef"=w92:T29)  [unwired: 8 in]
  n132 = global read "Flywheel_Globals.vi" "Flywheel_Right"() -> (w307:string)
  n133 = call <vilib>:"Spark MAX Set Output Advanced.vi"("error in (no error)"=w239, "Control Mode"=Spark_MAX_Control_Type."Percent VBus", "Setpoint"=0.0, "MotorControlDevRef"=w238) -> ("error out"=w311:errorcluster, "MotorControlDevRef"=w310:T29)  [unwired: 6 in]
  n134 = call <vilib>:"WPI_MotorControlRefNum Registry Set.vi"("error in (no error)"=w86, "refnum name"=w278, "MotorControlDevRef"=w87) -> ()  [unwired: 7 in, 2 out]
  n135 = call <vilib>:"Spark MAX Set Output Advanced.vi"("error in (no error)"=w242, "Control Mode"=Spark_MAX_Control_Type."Percent VBus", "Setpoint"=0.0, "MotorControlDevRef"=w243) -> ("error out"=w284:errorcluster, "MotorControlDevRef"=w309:T29)  [unwired: 6 in]
  n136 = call <vilib>:"Spark MAX Set PIDF Constants.vi"("error in"=w311, "PID Constants"=w5, "MotorControlDeviceRef"=w310) -> ("error out"=w105:errorcluster, "MotorControlDeviceRef"=w104:T29)  [unwired: 7 in]
  n137 = call <vilib>:"WPI_MotorControlRefNum Registry Set.vi"("error in (no error)"=w93, "refnum name"=w297, "MotorControlDevRef"=w92) -> ()  [unwired: 7 in, 2 out]
  n138 = call <vilib>:"WPI_MotorControlRefNum Registry Set.vi"("error in (no error)"=w97, "refnum name"=w298, "MotorControlDevRef"=w96) -> ()  [unwired: 7 in, 2 out]
  n139 = call <vilib>:"Spark MAX Set PIDF Constants.vi"("error in"=w284, "PID Constants"=w5, "MotorControlDeviceRef"=w309) -> ("error out"=w109:errorcluster, "MotorControlDeviceRef"=w108:T29)  [unwired: 7 in]
  n140 = call <vilib>:"Spark MAX Burn Flash.vi"("error in"=w105, "MotorControlDeviceRef"=w104) -> ("error out"=w102:errorcluster, "MotorControlDeviceRef"=w103:T29)  [unwired: 8 in]
  n141 = call <vilib>:"Spark MAX Burn Flash.vi"("error in"=w109, "MotorControlDeviceRef"=w108) -> ("error out"=w107:errorcluster, "MotorControlDeviceRef"=w106:T29)  [unwired: 8 in]
  n142 = call <vilib>:"WPI_MotorControlRefNum Registry Set.vi"("error in (no error)"=w102, "refnum name"=w328, "MotorControlDevRef"=w103) -> ()  [unwired: 7 in, 2 out]
  n143 = call <vilib>:"WPI_MotorControlRefNum Registry Set.vi"("error in (no error)"=w107, "refnum name"=w307, "MotorControlDevRef"=w106) -> ()  [unwired: 7 in, 2 out]
  n144 = disable-structure shown="Disabled" {
    frame Disabled {
      n145 = call <vilib>:"Spark MAX Configure Alternate Encoder.vi"("Inverted (F)"=TRUE, "Cycles per Revolution (4096)"=u32 34) -> ("error out"=w370:errorcluster, "MotorControlDeviceRef"=w369:T29)  [unwired: 8 in]
      n146 = call <vilib>:"Spark MAX Set Feedback Sensor Type.vi"("error in (no error)"=w370, "Sensor Type"=Spark_MAX_Sensor_Type."Alternate Encoder", "MotorControlDevRef"=w369) -> ()  [unwired: 7 in, 2 out]
    }
    frame Enabled {
    }
  }
  n147 = call <vilib>:"Spark MAX Open.vi"("Device Number"=u8 3) -> ("error out"=w110:errorcluster, "MotorControlDeviceRef"=w111:T29)  [unwired: 9 in]
  n148 = call <vilib>:"Spark MAX Set Current Limit.vi"("error in (no error)"=w110, "Current Limit A (100)"=sgl 30.0, "MotorControlDeviceRef in"=w111) -> ("error out"=w182:errorcluster, "MotorControlDeviceRef out"=w183:T29)  [unwired: 7 in]
  n149 = call <vilib>:"Spark MAX Set Motor Type.vi"("error in (no error)"=w182, "Motor Type"=Spark_MAX_Motor_Type."Brushless", "MotorControlDevRef"=w183) -> ("error out"=w234:errorcluster, "MotorControlDeviceRef"=w235:T29)  [unwired: 7 in]
  n150 = global read "Solenoid Globals.vi" "Hopper/Climb"() -> (w67:string)
  n151 = call <vilib>:"Spark MAX Set Idle Mode.vi"("error in (no error)"=w234, "Idle Mode"=Spark_MAX_Idle_Mode."Brake", "MotorControlDeviceRef in"=w235) -> ("error out"=w233:errorcluster, "MotorControlDeviceRef out"=w232:T29)  [unwired: 7 in]
  n152 = global read "Solenoid Globals.vi" "Compressor"() -> (w80:string)
  n153 = call <vilib>:"WPI_CompressorOpen.vi"("Pneumatics Control Module (0)"=u8 0) -> ("CompressorDevRef"=w64:T35, "error out"=w65:errorcluster)  [unwired: 13 in]
  n154 = call <vilib>:"Spark MAX Open.vi"("Device Number"=u8 10) -> ("error out"=w195:errorcluster, "MotorControlDeviceRef"=w196:T29)  [unwired: 9 in]
  n155 = call <vilib>:"Spark MAX Set Output Advanced.vi"("error in (no error)"=w233, "Control Mode"=Spark_MAX_Control_Type."Percent VBus", "Setpoint"=0.0, "MotorControlDevRef"=w232) -> ("error out"=w114:errorcluster, "MotorControlDevRef"=w115:T29)  [unwired: 6 in]
  n156 = global read "Turret_Globals.vi" "Turret_Spin"() -> (w326:string)
  n157 = call-poly <vilib>:"WPI_SolenoidOpen.vi"("Reverse Solenoid Channel"=WPI_SolenoidChannel."Solenoid 5", "Forward Solenoid Channel"=WPI_SolenoidChannel."Solenoid 4" ("Solenoid Channel"), "Pneumatics Control Module (0)"=u8 0) -> ("error out"=w69:errorcluster, "SolenoidDevRef"=w68:T36)  [unwired: 7 in]
  n158 = call <vilib>:"WPI_CompressorStart.vi"("error in (no error)"=w65, "CompressorDevRef"=w64) -> ("error out"=w62:errorcluster, "CompressorDevRef"=w63:T35)  [unwired: 8 in]
  n159 = call <vilib>:"Spark MAX Burn Flash.vi"("error in"=w114, "MotorControlDeviceRef"=w115) -> ("error out"=w113:errorcluster, "MotorControlDeviceRef"=w112:T29)  [unwired: 8 in]
  n160 = call <vilib>:"WPI_CompressorRefNum Registry Set.vi"("error in (no error)"=w62, "refnum name"=w80, "CompressorDevRef"=w63) -> ()  [unwired: 7 in, 2 out]
  n161 = call <vilib>:"WPI_SolenoidRefNum Registry Set.vi"("error in (no error)"=w69, "refnum name"=w67, "SolenoidDevRef"=w68) -> ()  [unwired: 7 in, 2 out]
  n162 = call <vilib>:"WPI_MotorControlRefNum Registry Set.vi"("error in (no error)"=w113, "refnum name"=w326, "MotorControlDevRef"=w112) -> ()  [unwired: 7 in, 2 out]
  n163 = global read "Solenoid Globals.vi" "Intake_Right_Extend"() -> (w77:string)
  n164 = global read "Solenoid Globals.vi" "Control_Panel_Pneumatic"() -> (w71:string)
  n165 = call <vilib>:"Spark MAX Open.vi"("Device Number"=u8 12) -> ("error out"=w172:errorcluster, "MotorControlDeviceRef"=w171:T29)  [unwired: 9 in]
  n166 = call <vilib>:"CTRE_Phoenix_TalonSRX_Open.vi"("Device Number"=u8 13) -> ("error out"=w273:errorcluster, "CAN Talon SRX Ref"=w272:T29)  [unwired: 9 in]
  n167 = call <vilib>:"Spark MAX Set Current Limit.vi"("error in (no error)"=w195, "Current Limit A (100)"=sgl 30.0, "MotorControlDeviceRef in"=w196) -> ("error out"=w198:errorcluster, "MotorControlDeviceRef out"=w197:T29)  [unwired: 7 in]
  n168 = call <vilib>:"CTRE_Phoenix_TalonSRX_Open.vi"("Device Number"=u8 14) -> ("error out"=w257:errorcluster, "CAN Talon SRX Ref"=w256:T29)  [unwired: 9 in]
  n169 = call <vilib>:"CTRE_Phoenix_TalonSRX_Open.vi"("Device Number"=u8 15) -> ("error out"=w258:errorcluster, "CAN Talon SRX Ref"=w259:T29)  [unwired: 9 in]
  n170 = call <vilib>:"Spark MAX Set Current Limit.vi"("error in (no error)"=w172, "Current Limit A (100)"=sgl 30.0, "MotorControlDeviceRef in"=w171) -> ("error out"=w169:errorcluster, "MotorControlDeviceRef out"=w170:T29)  [unwired: 7 in]
  n171 = call <vilib>:"CTRE_Phoenix_MotorControl_Set.vi"("error in (no error)"=w273, "Output"=0.0, "Control Mode"=w270, "PhoenixMotorControlDevRef"=w272) -> ("error out"=w268:errorcluster, "PhoenixMotorControlDevRef"=w267:T29)  [unwired: 6 in]
  n172 = call-poly <vilib>:"WPI_SolenoidOpen.vi"("Reverse Solenoid Channel"=WPI_SolenoidChannel."Solenoid 7", "Forward Solenoid Channel"=WPI_SolenoidChannel."Solenoid 6" ("Solenoid Channel"), "Pneumatics Control Module (0)"=u8 0) -> ("error out"=w73:errorcluster, "SolenoidDevRef"=w72:T36)  [unwired: 7 in]
  n173 = call-poly <vilib>:"WPI_SolenoidOpen.vi"("Reverse Solenoid Channel"=WPI_SolenoidChannel."Solenoid 1", "Forward Solenoid Channel"=WPI_SolenoidChannel."Solenoid 0" ("Solenoid Channel"), "Pneumatics Control Module (0)"=u8 0) -> ("error out"=w79:errorcluster, "SolenoidDevRef"=w78:T36)  [unwired: 7 in]
  n174 = call <vilib>:"WPI_SolenoidRefNum Registry Set.vi"("error in (no error)"=w79, "refnum name"=w77, "SolenoidDevRef"=w78) -> ()  [unwired: 7 in, 2 out]
  n175 = call <vilib>:"WPI_SolenoidRefNum Registry Set.vi"("error in (no error)"=w73, "refnum name"=w71, "SolenoidDevRef"=w72) -> ()  [unwired: 7 in, 2 out]
  n176 = call <vilib>:"Spark MAX Set Motor Type.vi"("error in (no error)"=w198, "Motor Type"=Spark_MAX_Motor_Type."Brushless", "MotorControlDevRef"=w197) -> ("error out"=w217:errorcluster, "MotorControlDeviceRef"=w216:T29)  [unwired: 7 in]
  n177 = call <vilib>:"CTRE_Phoenix_MotorControl_Set.vi"("error in (no error)"=w257, "Output"=0.0, "Control Mode"=w254, "PhoenixMotorControlDevRef"=w256) -> ("error out"=w252:errorcluster, "PhoenixMotorControlDevRef"=w251:T29)  [unwired: 6 in]
  n178 = global read "Climb_Globals.vi" "Climb_Elevator_Right"() -> (w266:string)
  n179 = call <vilib>:"CTRE_Phoenix_MotorControl_Set.vi"("error in (no error)"=w258, "Output"=0.0, "Control Mode"=w261, "PhoenixMotorControlDevRef"=w259) -> ("error out"=w263:errorcluster, "PhoenixMotorControlDevRef"=w264:T29)  [unwired: 6 in]
  n180 = global read "Climb_Globals.vi" "Climb_Elevator_Left"() -> (w250:string)
  n181 = call <vilib>:"Spark MAX Set Motor Type.vi"("error in (no error)"=w169, "Motor Type"=Spark_MAX_Motor_Type."Brushless", "MotorControlDevRef"=w170) -> ("error out"=w211:errorcluster, "MotorControlDeviceRef"=w208:T29)  [unwired: 7 in]
  n182 = call <vilib>:"Spark MAX Set Idle Mode.vi"("error in (no error)"=w217, "Idle Mode"=Spark_MAX_Idle_Mode."Brake", "MotorControlDeviceRef in"=w216) -> ("error out"=w215:errorcluster, "MotorControlDeviceRef out"=w214:T29)  [unwired: 7 in]
  n183 = call <vilib>:"CTRE_Phoenix_MotorControl_RefNumRegistrySet.vi"("error in (no error)"=w268, "refnum name"=w266, "PhoenixMotorControlDevRef"=w267) -> ()  [unwired: 7 in, 2 out]
  n184 = global read "Solenoid Globals.vi" "Intake_Left_Extend"() -> (w58:string)
  n185 = global read "Climb_Globals.vi" "Climb_Pivot"() -> (w274:string)
  n186 = call <vilib>:"CTRE_Phoenix_MotorControl_RefNumRegistrySet.vi"("error in (no error)"=w252, "refnum name"=w250, "PhoenixMotorControlDevRef"=w251) -> ()  [unwired: 7 in, 2 out]
  n187 = call <vilib>:"Spark MAX Set Idle Mode.vi"("error in (no error)"=w211, "Idle Mode"=Spark_MAX_Idle_Mode."Brake", "MotorControlDeviceRef in"=w208) -> ("error out"=w210:errorcluster, "MotorControlDeviceRef out"=w209:T29)  [unwired: 7 in]
  n188 = call <vilib>:"Spark MAX Set Output Advanced.vi"("error in (no error)"=w215, "Control Mode"=Spark_MAX_Control_Type."Percent VBus", "Setpoint"=0.0, "MotorControlDevRef"=w214) -> ("error out"=w285:errorcluster, "MotorControlDevRef"=w290:T29)  [unwired: 6 in]
  n189 = global read "Magazine_Globals.vi" "Magazine"() -> (w286:string)
  n190 = global read "Climb_Globals.vi" "Climb_Transverse"() -> (w265:string)
  n191 = call <vilib>:"Spark MAX Set Output Advanced.vi"("error in (no error)"=w210, "Control Mode"=Spark_MAX_Control_Type."Percent VBus", "Setpoint"=0.0, "MotorControlDevRef"=w209) -> ("error out"=w82:errorcluster, "MotorControlDevRef"=w83:T29)  [unwired: 6 in]
  n192 = call <vilib>:"Spark MAX Set PIDF Constants.vi"("error in"=w285, "PID Constants"=T4 {"P Gain"=0.0001, "I Gain"=0.0, "D Gain"=0.0, "F Gain"=0.5, "I Zone"=0.0, "Min Output"=-1.0, "Max Output"=1.0}, "MotorControlDeviceRef"=w290) -> ("error out"=w98:errorcluster, "MotorControlDeviceRef"=w101:T29)  [unwired: 7 in]
  n193 = call <vilib>:"CTRE_Phoenix_MotorControl_RefNumRegistrySet.vi"("error in (no error)"=w263, "refnum name"=w265, "PhoenixMotorControlDevRef"=w264) -> ()  [unwired: 7 in, 2 out]
  n194 = call-poly <vilib>:"WPI_SolenoidOpen.vi"("Reverse Solenoid Channel"=WPI_SolenoidChannel."Solenoid 3", "Forward Solenoid Channel"=WPI_SolenoidChannel."Solenoid 2" ("Solenoid Channel"), "Pneumatics Control Module (0)"=u8 0) -> ("error out"=w56:errorcluster, "SolenoidDevRef"=w57:T36)  [unwired: 7 in]
  n195 = call <vilib>:"Spark MAX Burn Flash.vi"("error in"=w82, "MotorControlDeviceRef"=w83) -> ("error out"=w84:errorcluster, "MotorControlDeviceRef"=w85:T29)  [unwired: 8 in]
  n196 = call <vilib>:"Spark MAX Burn Flash.vi"("error in"=w98, "MotorControlDeviceRef"=w101) -> ("error out"=w99:errorcluster, "MotorControlDeviceRef"=w100:T29)  [unwired: 8 in]
  n197 = call <vilib>:"WPI_SolenoidRefNum Registry Set.vi"("error in (no error)"=w56, "refnum name"=w58, "SolenoidDevRef"=w57) -> ()  [unwired: 7 in, 2 out]
  n198 = call <vilib>:"WPI_MotorControlRefNum Registry Set.vi"("error in (no error)"=w99, "refnum name"=w286, "MotorControlDevRef"=w100) -> ()  [unwired: 7 in, 2 out]
  n199 = call <vilib>:"WPI_MotorControlRefNum Registry Set.vi"("error in (no error)"=w84, "refnum name"=w274, "MotorControlDevRef"=w85) -> ()  [unwired: 7 in, 2 out]
  "error out" <- "error in"
